vi "Read_BSA_No_of_points.vi"(3 "error in (no error)":errorcluster, 6 "GPIB Address":string) -> (0 "error out":errorcluster, 1 "No of samples":i32)   [LabVIEW 2010]
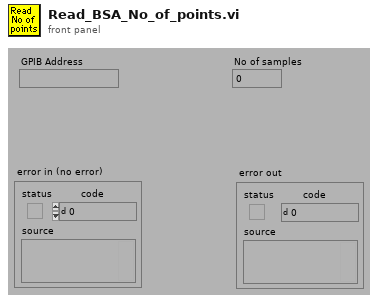
[diagram p1: front panel]
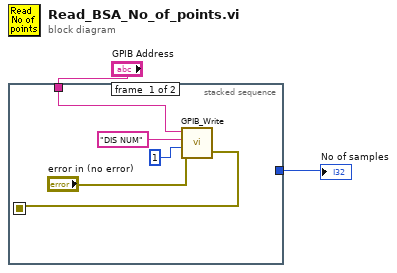
[diagram p0: block diagram]
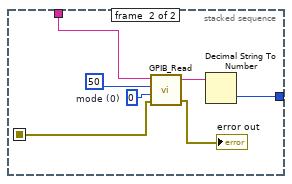
[diagram p2: hidden frame]
diagram:
  n1 = stacked-sequence {
    seq-local: [w4 _] -> [_ w10]
    tunnel: "GPIB Address" -> [w6 w14]
    tunnel: [_ w9] -> w1
    frame #0 {
      n2 = call "GPIB_Write.vi"("address string"=w6, "data In"="DIS NUM", "mode (0)"=i16 1, "error in"="error in (no error)") -> ("error out"=w4:errorcluster)  [unwired: 1 in, 1 out]
    }
    frame #1 {
      w12 = i16 0  # mode (0)
      n3 = call "GPIB_Read.vi"("address string"=w14, "byte count"=50, "mode (0)"=w12, "error in"=w10) -> ("data Out"=w13:string, "error out"=→"error out":errorcluster)  [unwired: 1 in, 1 out]
      n4 = Decimal String To Number(string=w13) -> (number=w9:i32)  [unwired: 3 out]
    }
  }
  "No of samples" <- w1
